vi "Graph function.vi"(5 "# of iterations":i32, 7 "Starting x value":i32, 11 "Function Parameters":cluster{"a":dbl, "b":dbl, "c":dbl, "d":dbl}) -> (2 "XY Data":cluster{i32[], dbl[]})   [LabVIEW 2010]
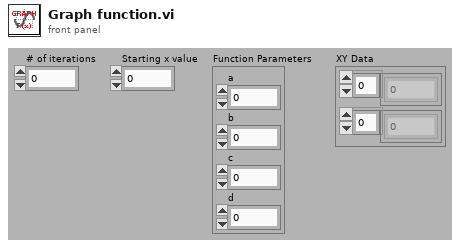
[diagram p1: front panel]
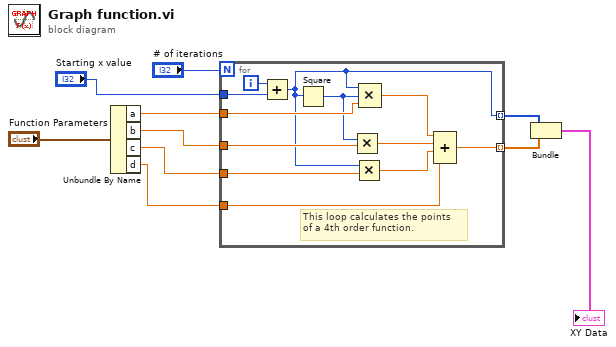
[diagram p0: block diagram]
diagram:
  n1 = Unbundle By Name("Function Parameters") -> ("a"=w7:dbl, "b"=w8:dbl, "c"=w9:dbl, "d"=w10:dbl)
  n2 = for {
    N: "# of iterations" -> [_]
    tunnel: w7 -> [w22]
    tunnel: w8 -> [w20]
    tunnel: w9 -> [w19]
    tunnel: w10 -> [w15]
    tunnel: [w14] -> w1 mode=indexing
    tunnel: [w13] -> w2 mode=indexing
    tunnel: "Starting x value" -> [w12]
    i -> [w11]
    # "This loop calculates the points \nof a 4th order function."
    n3 = Add(x=w11, y=w12) -> (x+y=w13:i32)
    n4 = Square(x=w13) -> (x^2=w21:i32)
    n5 = Multiply(x=w21, y=w20) -> (x*y=w17:dbl)
    n6 = Multiply(x=w13, y=w19) -> (x*y=w18:dbl)
    n7 = Compound Arithmetic op=MULTIPLY(w13, w21, w22) -> (w16:dbl)
    n8 = Compound Arithmetic op=ADD(w16, w17, w18, w15) -> (w14:dbl)
  }
  n9 = Bundle(w2, w1) -> (→"XY Data":cluster{i32[], dbl[]})  [unwired: 1 in]
